vi "倒计时.vi"(10 "超限时间":dbl=12.0 format="%0.8f") -> (1 "倒计时":dbl, 2 "Time has Elapsed":bool)   [LabVIEW 2015]
panel:
  out "Elapsed Time":dbl format="%0.2f"
  out "error out":errorcluster
  in  "error in (no error)":errorcluster
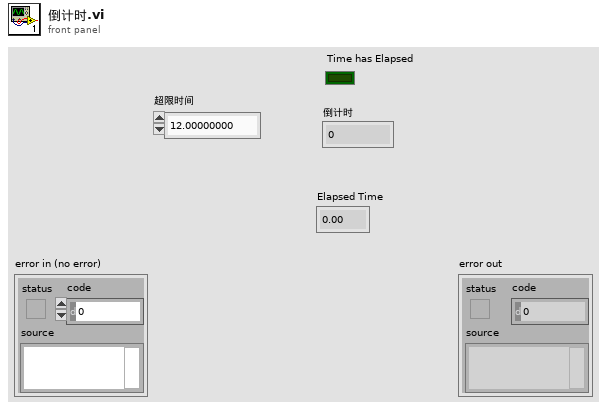
[diagram p1: front panel]
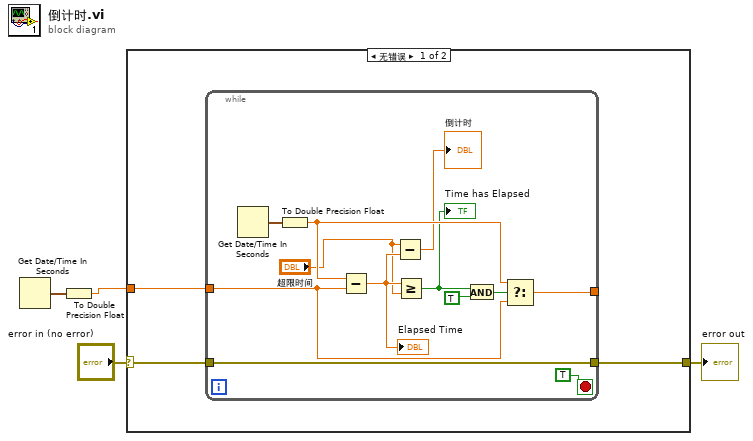
[diagram p0: block diagram]
diagram:
  n1 = Get Date/Time In Seconds() -> (seconds since 1Jan1904=w2:timestamp)
  n2 = To Double Precision Float(number=w2) -> (double precision float=w1:dbl)
  n3 = case shown="无错误" "error in (no error)" {
    selector: "error in (no error)" -> [w7 w20]
    tunnel: [w6 w20] -> w3
    tunnel: w1 -> [w5 _]
    frame No Error {
      n4 = while {
        tunnel: w5 -> [w10]
        tunnel: [w11] -> _
        tunnel: w7 -> [w9]
        tunnel: [w9] -> w6
        stop <- TRUE stop-if-true
        n5 = Get Date/Time In Seconds() -> (seconds since 1Jan1904=w16:timestamp)
        n6 = To Double Precision Float(number=w16) -> (double precision float=w15:dbl)
        n7 = Subtract(x=w15, y=w10) -> (x-y=w14:dbl)
        "Elapsed Time" <- w14
        n8 = Subtract(x="超限时间", y=w14) -> (x-y=→"倒计时":dbl)
        n9 = Greater Or Equal?(x=w14, y="超限时间") -> (x >= y?=w13:bool)
        "Time has Elapsed" <- w13
        n10 = And(x=w13, y=TRUE ("Auto Reset")) -> (x .and. y?=w17:bool)
        n11 = Select(t=w15, s=w17, f=w10) -> (s? t:f=w11:dbl)
      }
    }
    frame Error {
    }
  }
  "error out" <- w3
